vi "LVClass_Camera set background.vi"(0 "Camera in":refnum<class "Camera.lvclass">, 5 "Image.lvclass":refnum<class "Image.lvclass">, 11 "error in (no error)":errorcluster) -> (4 "Camera out":refnum<class "Camera.lvclass">, 15 "error out":errorcluster)   [LabVIEW 2020, in "Camera.lvclass"]
doc: "Set Camera background image. Image with substracted background can be\nretrieved using the Imop_Camera_GetLastImage function with remove_background_c\n= 1.\n\n<B>CameraIn</B> : Camera object.\n<B>CameraOut</B> : Camera object.\n<B>bg_Image</B> : Background image."
uses:
  Camera.lvclass
  Image.lvclass
  Camera.lvclass/Camera.ctl
  LVClass_Image read Image Compat ptr.vi
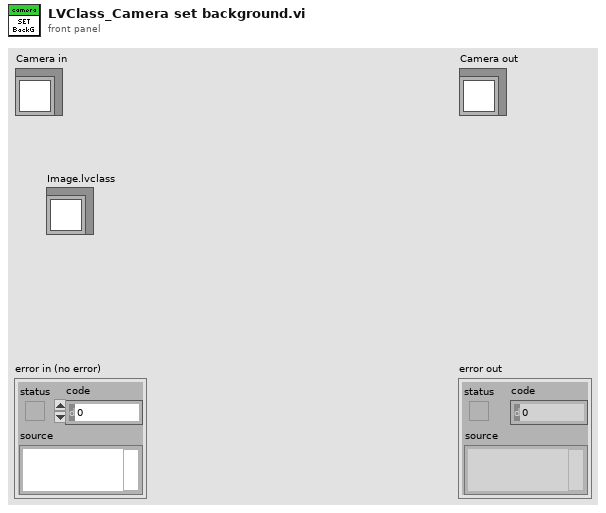
[diagram p1: front panel]
types:
  T1 = typedef "ClassID.ctl" = i64
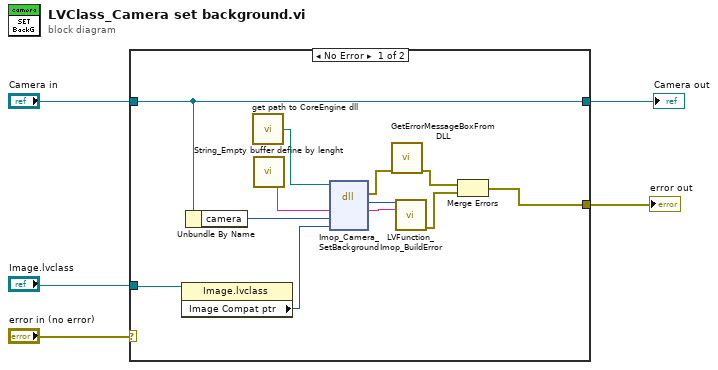
[diagram p0: block diagram]
diagram:
  n1 = case shown="No Error" "error in (no error)" {
    selector: "error in (no error)" -> [_ w19]
    tunnel: [w6 w19] -> w4
    tunnel: [w13 w18] -> w2
    tunnel: "Camera in" -> [w13 w18]
    tunnel: "Image.lvclass" -> [w11 _]
    frame No Error {
      n2 = property class="Image.lvclass"(reference=w11) -> ("Image Compat ptr"=w12:T1)  [unwired: 1 in, 2 out]
      n3 = Unbundle By Name(w13) -> ("camera"=w14:T1)
      n4 = call "get path to CoreEngine dll.vi"() -> ("path to c_interface_vc100.dll"=w10:path)  [unwired: 12 in, 3 out]
      n5 = call "String_Empty buffer define by lenght.vi"() -> ("Empty buffer"=w17:string)  [unwired: 1 in]
      n6 = dll-call lib="D:/2_trunk/Soft_haso/ImOpCoreEngine4_LV2011/DLLs/ImopEngine4_vc100.dll" fn="Imop_Camera_SetBackground"(path in=w10, "message"=w17, "camera"=w14, "HASO_image"=w12) -> (error out=w9:errorcluster, "return type"=w16:i32, "message"=w15:string)  [unwired: 4 in, 1 out]
      n7 = call "GetErrorMessageBoxFromDLL.vi"("error IN"=w9) -> ("error OUT"=w8:errorcluster)  [unwired: 10 in]
      n8 = call "LVFunction_Imop_BuildError.vi"("code"=w16, "String to Prepend to source (\"\")"=w15) -> ("error out"=w7:errorcluster)  [unwired: 13 in]
      n9 = Merge Errors(w8, w7) -> (w6:errorcluster)
    }
    frame Error {
    }
  }
  "error out" <- w4
  "Camera out" <- w2
